vi "Object orientation + stepper control.vi"() -> ()   [LabVIEW 2018]
uses:
  Underlying VI's/I2C Master VI/I2C_MASTER_WRITE_NEW Type Def.ctl
  <vilib>/userdefined/High Color/IMAQdx.ctl
  Underlying VI's/Webcam FGV Low level ver/State control.ctl
panel:
  in  "ENA":bool
  in  "Arduino mode":T1
  out "Corrected stepper":u8
  out "error out":errorcluster
  out "Error out":errorcluster
  in  "stop":bool
  out "Image":T2(plugin-control)
  out "Object Center Coordinates":cluster{"x":sgl, "y":sgl}
  out "Object detection cluster":T3
  in  "Mode":enum16{"Ball", "Soap", "Gel", "Pipe", "None"}(ring)
  # "Save me pls"
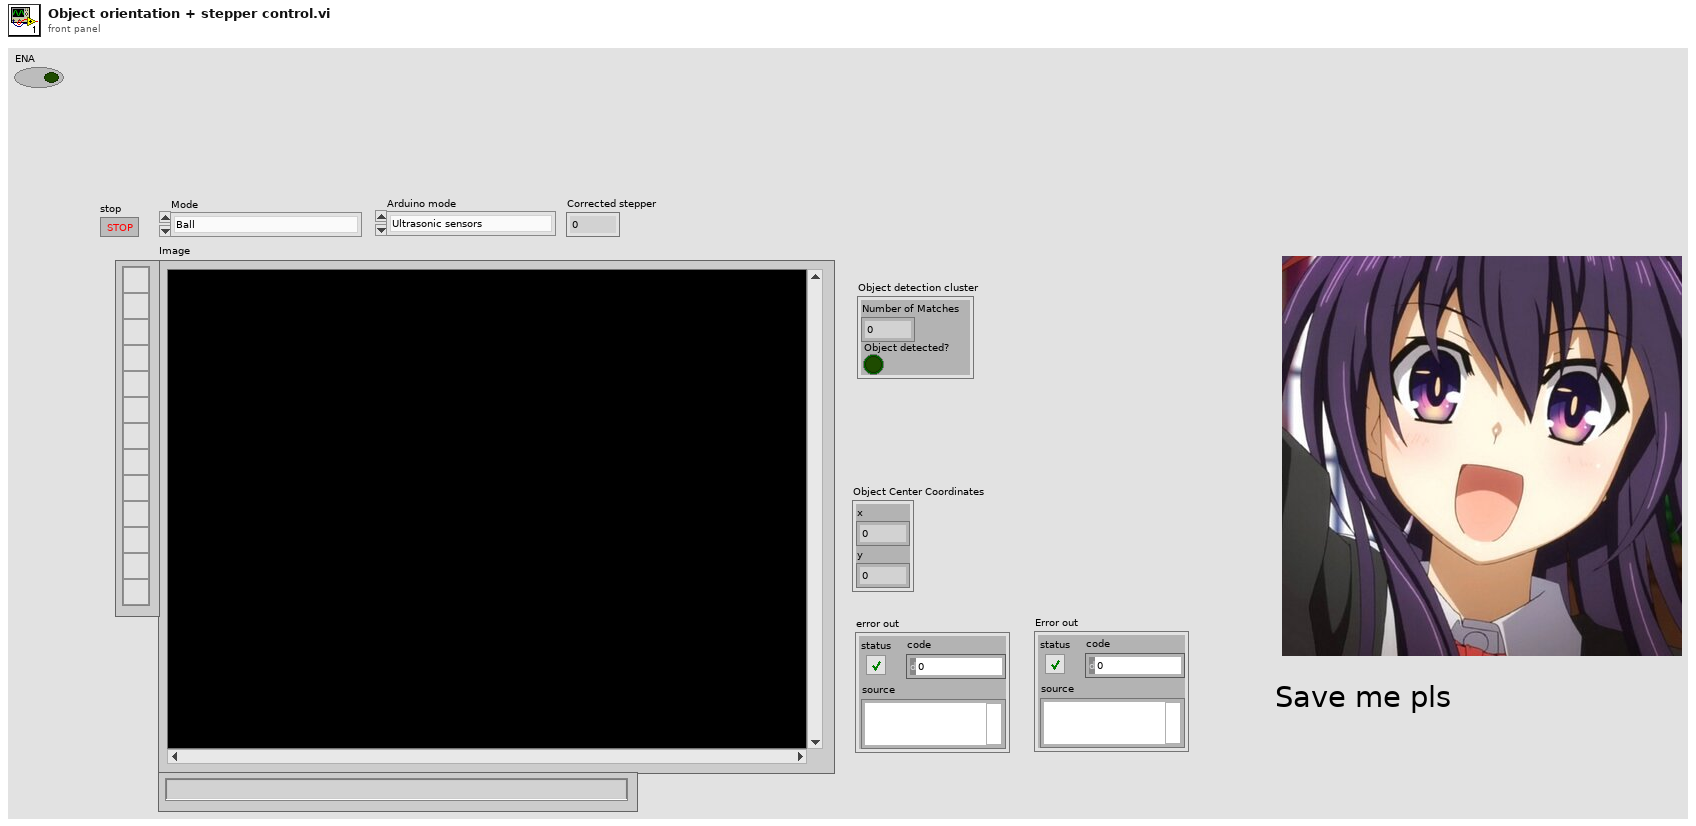
[diagram p1: front panel]
types:
  T1 = typedef "I2C_MASTER_WRITE_NEW Type Def.ctl" = enum16{"Ultrasonic sensors", "Stepper origin", "zStepper 13.3k", "zStepper 13k", "zStepper 12k", "zStepper 11k", "zStepper 10k", "zStepper 9k", "zStepper 8k", "zStepper 7k", "zStepper 6k", "zStepper 5k", "zStepper 4k", "zStepper 3k", "zStepper 2k", "zStepper 1k", "zStepper 900", "zStepper 800", "zStepper 700", "zStepper 600", "zStepper 500", "zStepper 400", "zStepper 300", "zStepper 200", "zStepper 100", "zStepper 0", "yStepper control", "Open Claw", "Close Claw", "Soft Reset"}
  T2 = typedef "IMAQ Image.ctl" = refnum<image>
  T3 = cluster{"Number of Matches":i32, "Object detected?":bool}
  T4 = typedef "State control.ctl" = enum16{"Initialise", "Start camera", "Continuous Acquisition ", "Stop camera", "Dispose all"}
  T5 = typedef "IMAQdx.ctl" = refnum<k21>
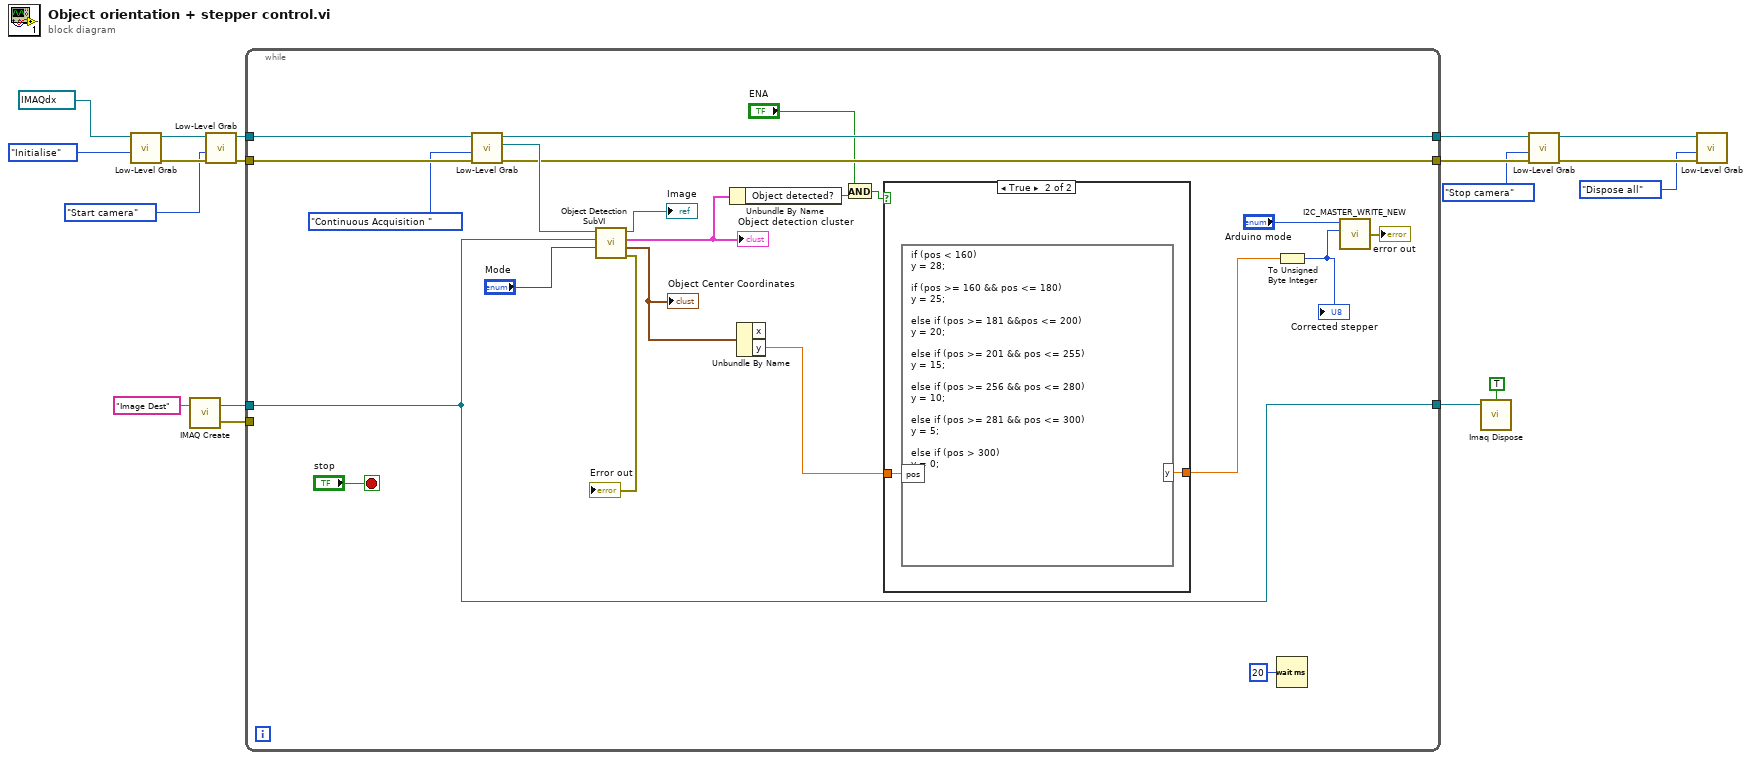
[diagram p0: block diagram]
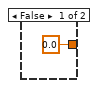
[diagram p2: hidden frame]
diagram:
  n1 = call "Low-Level Grab.vi"("States"=State_control."Initialise", "Session In"=T5 "cam0") -> ("error out"=w17:errorcluster, "Session Out"=w18:T5)  [unwired: 7 in, 1 out]
  n2 = call "IMAQ Create"("Image Name"="Image Dest") -> ("New Image"=w5:T2, "error out"=w2:errorcluster)  [unwired: 4 in]
  n3 = call "Low-Level Grab.vi"("error in (no error)"=w17, "States"=State_control."Start camera", "Session In"=w18) -> ("error out"=w13:errorcluster, "Session Out"=w12:T5)  [unwired: 6 in, 1 out]
  n4 = while {
    tunnel: w13 -> [w39]
    tunnel: w12 -> [w40]
    tunnel: [w36] -> w11
    tunnel: [w35] -> w10
    tunnel: w5 -> [w30]
    tunnel: [w30] -> w3
    tunnel: w2 -> [_]
    stop <- "stop" stop-if-true
    n5 = call "Low-Level Grab.vi"("error in (no error)"=w39, "States"=State_control."Continuous Acquisition ", "Session In"=w40) -> ("error out"=w35:errorcluster, "Image Out"=w37:T2, "Session Out"=w36:T5)  [unwired: 6 in]
    n6 = call "Object Detection SubVI.vi"("Mode"="Mode", "Image Dest"=w30, "Image in"=w37) -> ("Error out"=→"Error out":errorcluster, "Object Center Coordinates"=w28:cluster{"x":sgl, "y":sgl}, "Object detection cluster"=w22:T3, "Image Out"=→"Image":T2)  [unwired: 1 in]
    "Object detection cluster" <- w22
    "Object Center Coordinates" <- w28
    n7 = Unbundle By Name(w22) -> ("Object detected?"=w21:bool)
    n8 = Unbundle By Name(w28) -> ("y"=w24:sgl)  [unwired: 1 out]
    n9 = And(x="ENA", y=w21) -> (x .and. y?=w19:bool)
    n10 = case shown="True" w19 {
      tunnel: w24 -> [_ w43]
      tunnel: [0.0 ("y") w42] -> w23
      frame False {
      }
      frame True {
        n11 = formula code="if (pos < 160)\ny = 28;\n\nif (pos >= 160 && pos <= 180)\ny = 25;\n\nelse if (pos >= 181 &&pos <= 200) \ny = 20;\n\nelse if (pos >= 201 && pos <= 255)\ny = 15;\n\nelse if (pos >= 256 && pos <= 280)\ny = 10;\n\nelse if (pos >= 281 && pos <= 300)\ny = 5;\n\nelse if (pos > 300)\ny = 0;"("pos"=w43) -> ("y"=w42:dbl)
      }
    }
    n12 = To Unsigned Byte Integer(number=w23) -> (unsigned 8bit integer=w26:u8)
    "Corrected stepper" <- w26
    n13 = Wait (ms)(milliseconds to wait=u32 20) -> ()  [unwired: 1 out]
    n14 = call "I2C_MASTER_WRITE_NEW.vi"("y Stepper value"=w26, "Arduino mode"="Arduino mode") -> ("error out"=→"error out":errorcluster)  [unwired: 2 in]
  }
  n15 = call "Imaq Dispose"("All Images? (No)"=TRUE, "Image"=w3) -> ()  [unwired: 4 in, 1 out]
  n16 = call "Low-Level Grab.vi"("error in (no error)"=w10, "States"=State_control."Stop camera", "Session In"=w11) -> ("error out"=w8:errorcluster, "Session Out"=w9:T5)  [unwired: 6 in, 1 out]
  n17 = call "Low-Level Grab.vi"("error in (no error)"=w8, "States"=State_control."Dispose all", "Session In"=w9) -> ()  [unwired: 6 in, 3 out]
